vi "execute_value_write_policy.vi"(8 "error in (no error)":errorcluster, 9 "Publish Time":timestamp, 10 "New Topic Value":variant, 11 "TimedAverageSubscription In":refnum<class "TimedAverageSubscription.lvclass">) -> (0 "error out":errorcluster, 3 "TimedAverageSubscription Out":refnum<class "TimedAverageSubscription.lvclass">)   [LabVIEW 2015, in "SubscriptionPolicy.lvlib" / "TimedAverageSubscription.lvclass"]
uses:
  TimedAverageSubscription.lvclass
  TimedAverageSubscription.lvclass/TimedAverageSubscription.ctl
  IMediator/ISubscriptionPolicy/ISubscriptionPolicy.lvclass/ISubscriptionPolicy.ctl
  IMediator/ITransport/ITransport.lvclass
  IMediator/ISubscriptionPolicy/ISubscriptionPolicy.lvclass
  Components/TimedAverageBuffer/TimedAverageBuffer.lvclass
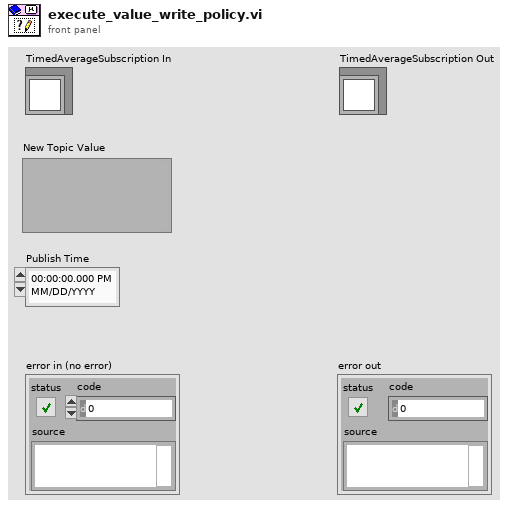
[diagram p1: front panel]
types:
  T1 = typedef "TimedAverageBuffer.lvlib/TimedAverageBuffer.lvclass/TimedAverageBuffer Reference.ctl" = refnum<data-value>
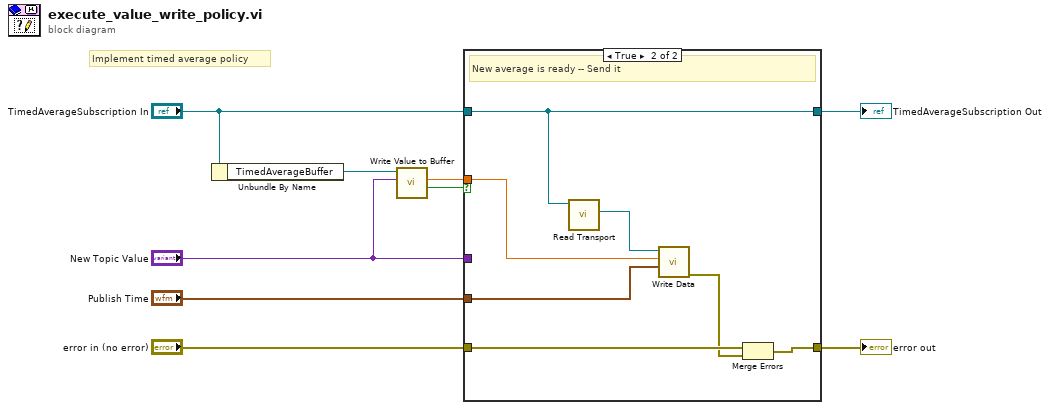
[diagram p0: block diagram]
diagram:
  # "Implement timed average policy"
  n1 = Unbundle By Name("TimedAverageSubscription In") -> ("TimedAverageBuffer"=w4:T1)
  n2 = call "Write Value to Buffer.vi"("Value"="New Topic Value", "Timed Average Buffer"=w4) -> ("New Average Ready?"=w2:bool, "Average"=w1:dbl)  [unwired: 6 in, 2 out]
  n3 = case shown="True" w2 {
    tunnel: "New Topic Value" -> [_ _]
    tunnel: "Publish Time" -> [_ w18]
    tunnel: "error in (no error)" -> [w10 w17]
    tunnel: [w10 w16] -> w7
    tunnel: "TimedAverageSubscription In" -> [w11 w13]
    tunnel: [w11 w13] -> w5
    tunnel: w1 -> [_ w12]
    frame False {
      # "No new average -- Do nothing"
    }
    frame True {
      # "New average is ready -- Send it"
      n4 = call "Read Transport.vi"("ISubscriptionPolicy in"=w13) -> ("Transport"=w14:refnum<class "ITransport.lvclass">)  [unwired: 10 in]
      n5 = call-dynamic "Write Data.vi"("Publication Time"=w18, "Value"=w12, "ITransport in"=w14) -> ("error out"=w15:errorcluster)  [unwired: 7 in, 1 out]
      n6 = Merge Errors(w17, w15) -> (w16:errorcluster)
    }
  }
  "error out" <- w7
  "TimedAverageSubscription Out" <- w5
